vi "FPGA VI with RMS.vi"() -> ()   [LabVIEW 2023]
uses:
  <vilib>/Platform/TimedLoop/XDataNode/timing_clust.ctl
  <vilib>/Platform/TimedLoop/XDataNode/nitl_modes.ctl
  <vilib>/Platform/TimedLoop/XDataNode/wakeup.ctl
  <vilib>/rvi/FXPMathLib/basic elements/FxpIntAccumulator/subVIs/nifxpmath_IntAccumulator_SimConfig.ctl
  <vilib>/rvi/FXPMathLib/FxpSqrt/subVIs/nifxpmath_Sqrt_SimConfig.ctl
  <vilib>/fxp/LVFixedPointOverflowPolicyTypeDef.ctl
  <vilib>/rvi/Emulation/niFpgaGetClockAttributes.vi
  <vilib>/rvi/Emulation/niFpgaSctlEmulationGetInTimedLoop.vi
  <vilib>/rvi/Emulation/niFpgaEmulationReportErrorSimple.vi
  <vilib>/rvi/eio/common/nirviEmuTemplateMethod_errors.vi
  <vilib>/rvi/Emulation/niFpgaCriticalErrorInLSC.vi
  <vilib>/rvi/Analysis/common/codeGenErrors/XNode/niFpgaXNodeCodeGenErrorHandle.vi
  <vilib>/rvi/Analysis/measure/dc-rms/templates/niFPGA Hanning LUT subVI.vi
  <vilib>/rvi/Analysis/measure/dc-rms/templates/niFPGA Convert LUT Val to Hanning Coeff.vi
  <vilib>/rvi/FXPMathLib/basic elements/FxpIntAccumulator/simVIs/DllFxpIntAccumulator_sub.vi
  <vilib>/rvi/FXPMathLib/FxpSqrt/simVIs/DllSqrtTemp_sub.vi
  <vilib>/eio/utilities/niEioResolveVilibRelativePath.vi
  <vilib>/rvi/interface/RandomDataEmulation/niFpgaRandomDataHandleErrors.vi
  <vilib>/eio/EIONode/EIONode.xnode
  <vilib>/rvi/Analysis/measure/dc-rms/XNode/niFpgaDC-RMS.xnode
  <vilib>/Platform/TimedLoop/XDataNode/XDataNode.xnode
  <vilib>/rvi/FXPMathLib/basic elements/FxpIntAccumulator/XNode/nifxpmath_IntAccumulator.xnode
  <vilib>/rvi/FXPMathLib/FxpMul/XNode/nifxpmath_Multiplier.xnode
  <vilib>/rvi/FXPMathLib/FxpSqrt/XNode/nifxpmath_Sqrt.xnode
  <vilib>/rvi/DataTransferAndStorage/Container/XNode/niFpgaContainer.xnode
  <vilib>/rvi/interface/RandomDataEmulation/nirviRandomDataFpgaReadWriteTemplate.vi
  <vilib>/Platform/TimedLoop/XDataNode/XDNodeRunTimeDep.lvlib
  <vilib>/rvi/FXPMathLib/sim/FxpSim.dll
panel:
  in  "Count(Ticks)":u32=25
  out "Loop Timer":u32
  out "Timed Out?":bool
  out "RMS":fxp<+,27,5>
  out "RMS Waveform":sgl(graph)
  out "Waveform Chart 2":sgl(graph)
  in  "Frequency":u64=10000
  out "I/P (periods/tick)":fxp<+,32,0>=2.4999957531690598e-05
  # "Loop 2 (Signal From the Tuning Fork)"
  # "Loop 1 (Signal to the Tuning Fork)"
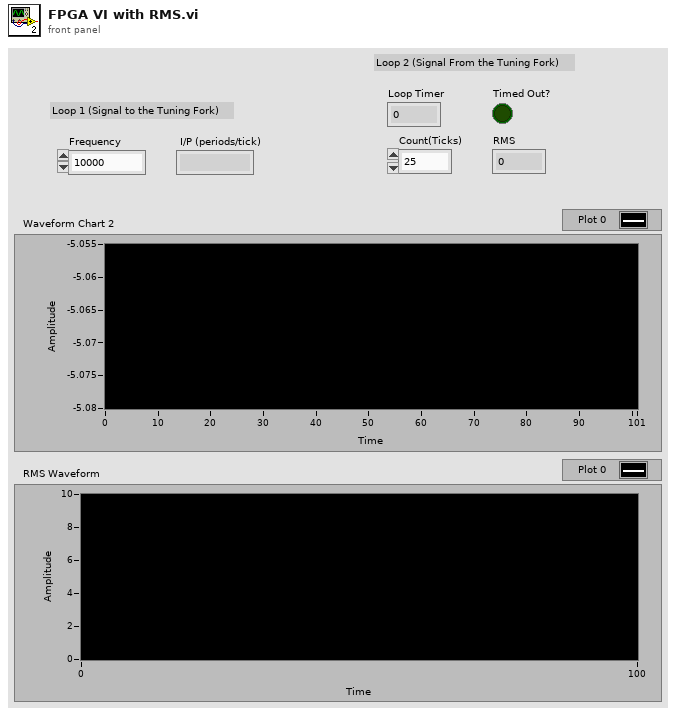
[diagram p1: front panel]
types:
  T1 = typedef "XDNodeRunTimeDep.lvlib/timing_clust.ctl" = cluster{"Expected End [f-1]":u64, "Actual End [f-1]":u64, "Finished Late? [f-1]":bool, "Expected End [i-1]":u64, "Actual End [i-1]":u64, "Finished Late? [i-1]":bool, "Expected Start [i]":u64, "Actual Start [i]":u64, "Expected Start [f]":u64, "Actual Start [f]":u64, "Source Name":string, "Structure Name":string, "Period":i64, "Deadline":i64, "Offset":i64, "Start":i64, "Priority":i32, "Timeout":i32, "Mode":T2, "Wakeup Reason":T3, "Error":errorcluster, "Source Type":string, "Secondary Source Type":string, "Global End Time":u64, "Global Start Time":u64, "Frame Duration":u64, "Iteration Duration":u64, "Assigned CPU":i32, "I/O Scan Engine Mode":u32}
  T2 = typedef "XDNodeRunTimeDep.lvlib/nitl_modes.ctl" = enum32{"No Change", "Process missed periods, maintain original phase", "Discard missed periods, maintain original phase", "Process missed periods, ignore original phase", "Discard missed periods, ignore original phase"}
  T3 = typedef "XDNodeRunTimeDep.lvlib/wakeup.ctl" = enum32{"Normal", "Aborted", "Asynchronous wakeup", "Timing source error", "Timed loop error", "Timeout"}
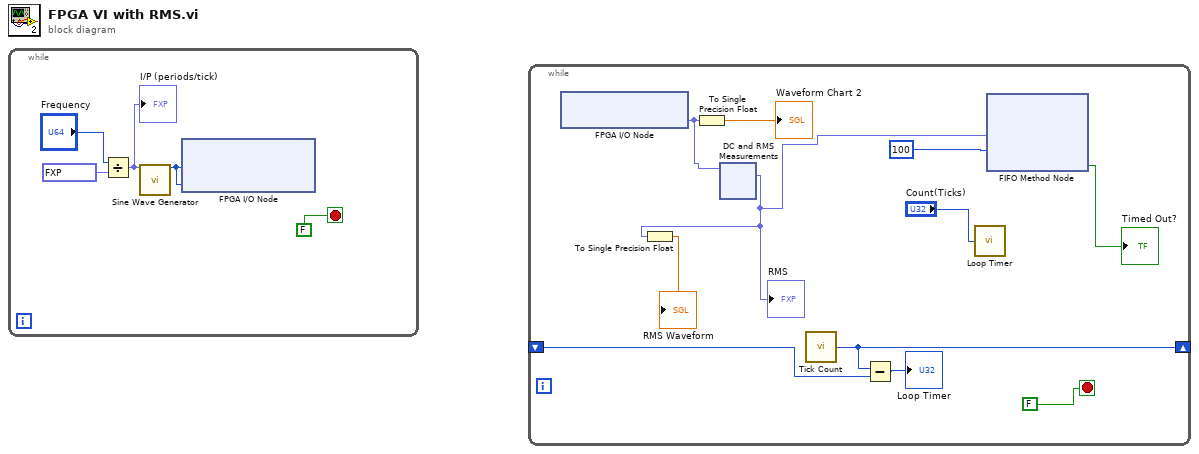
[diagram p0: block diagram]
diagram:
  n1 = while {
    stop <- FALSE stop-if-true
    n2 = Divide(x="Frequency", y=fxp<+,17,26> 40000000.0) -> (x/y=w3:fxp<+,64,39>)
    "I/P (periods/tick)" <- w3
    n3 = call "Sine Wave Generator"("frequency (periods/tick)"=w3) -> ("sine out"=w2:i16)  [unwired: 14 in]
    n4 = xnode "FPGA I/O Node"("Connector0/AO6"=w2, "Connector0/AO7"=w2) -> ()  [unwired: 2 in, 2 out]
  }
  n5 = while {
    shift-right: [w12] -> _
    shift-left: _ -> [w11]
    stop <- FALSE stop-if-true
    n6 = xnode "FPGA I/O Node"() -> ("Connector0/AI1"=w9:fxp<+/-,27,5>)  [unwired: 1 in, 1 out]
    n7 = To Single Precision Float(number=w9) -> (single precision float=→"Waveform Chart 2":sgl)
    n8 = xnode "DC and RMS Measurements"("input data"=w9) -> ("RMS"=w8:fxp<+,27,5>)  [unwired: 1 in, 1 out]
    "RMS" <- w8
    n9 = To Single Precision Float(number=w8) -> (single precision float=→"RMS Waveform":sgl)
    n10 = call "Tick Count"() -> ("Tick Count(Ticks)"=w12:u32)
    n11 = Subtract(x=w12, y=w11) -> (x-y=→"Loop Timer":u32)
    n12 = call "Loop Timer"("Count(Ticks)"="Count(Ticks)") -> ()  [unwired: 1 out]
    n13 = xnode ("FIFO Method Node")("Element"=w8, "Timeout"=100) -> ("Timed Out?"=→"Timed Out?":bool)  [unwired: 1 in, 1 out]
  }
